vi "ELVIS III v1.0 Reserve Channel List.vi"(7 "Allow multiple opens?":bool, 8 "error in (no error)":errorcluster, 10 "Channel Reservation List":T1, 11 "Owner":string) -> (0 "error out":errorcluster)   [LabVIEW 2021]
uses:
  <vilib>/myRIO/Common/Instrument Driver Framework/ELVIS III v1.0/Resource Manager/typedefs/ELVIS III v1.0 Channel Reservation List.ctl
  <vilib>/myRIO/Common/Instrument Driver Framework/ELVIS III v1.0/Resource Manager/typedefs/ELVIS III v1.0 Channel Reservation Info.ctl
  <vilib>/myRIO/Common/Instrument Driver Framework/ELVIS III v1.0/Resource Manager/typedefs/ELVIS III v1.0 Connector List.ctl
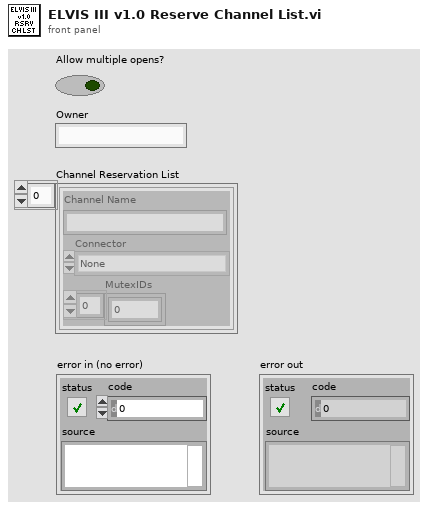
[diagram p1: front panel]
types:
  T1 = typedef "ELVIS III v1.0 Channel Reservation List.ctl" = T2[]
  T2 = typedef "ELVIS III v1.0 Channel Reservation Info.ctl" = cluster{"Channel Name":string, "Connector":T3, "MutexIDs":u32[]}
  T3 = typedef "ELVIS III v1.0 Connector List.ctl" = enum32{"None", "ConnectorA", "ConnectorB"}
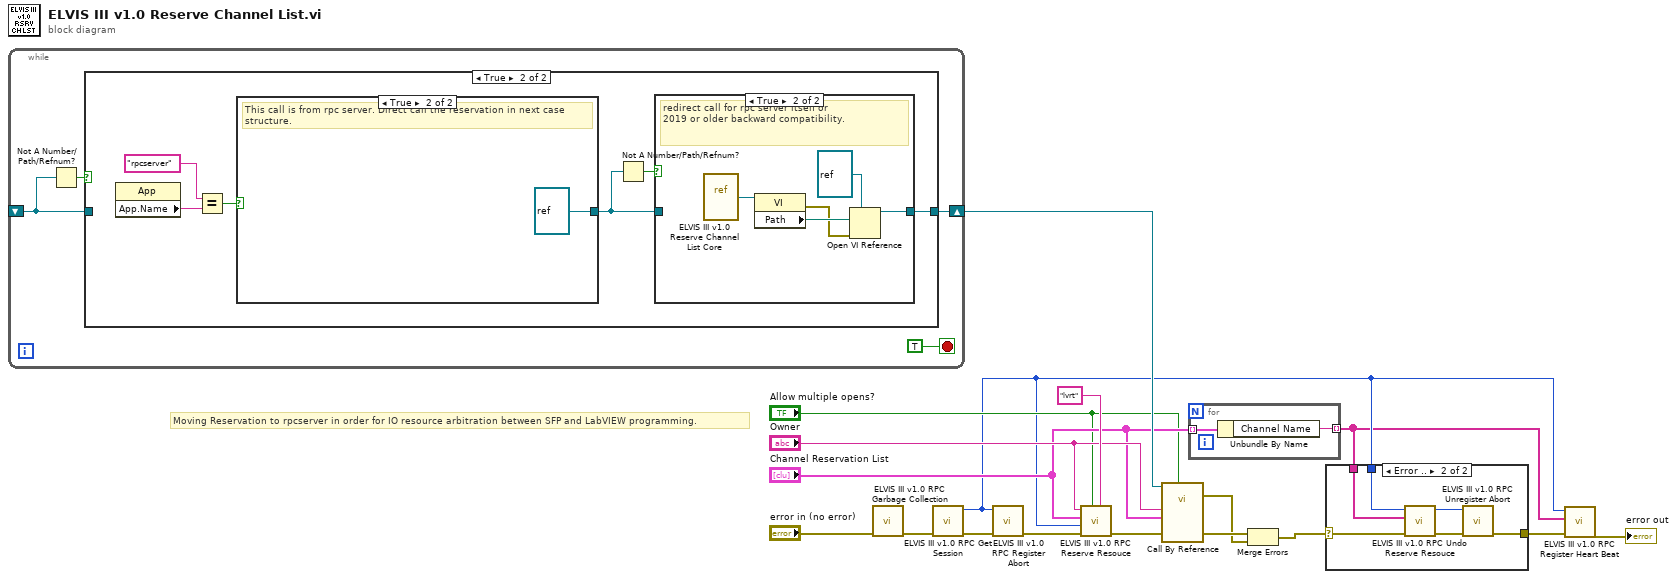
[diagram p0: block diagram]
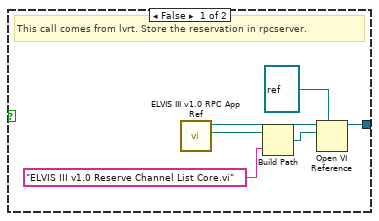
[diagram p5: hidden frame]
diagram:
  # "Moving Reservation to rpcserver in order for IO resource arbitration between SFP and LabVIEW programming."
  n1 = while {
    shift-right: [w21] -> w17
    shift-left: _ -> [w18]
    stop <- TRUE stop-if-true
    n2 = Not A Number/Path/Refnum?(number/path/refnum=w18) -> (NaN/Path/Refnum?=w19:bool)
    n3 = case shown="True" w19 {
      tunnel: [w22 w23] -> w21
      tunnel: w18 -> [w22 _]
      frame False {
      }
      frame True {
        n4 = property class="App"() -> ("App.Name"=w28:string)  [unwired: 2 in, 2 out]
        n5 = Equal?(x="rpcserver" ("Application:Name"), y=w28) -> (x = y?=w27:bool)
        n6 = case shown="True" w27 {
          tunnel: [w39 refnum<vi> refnum ("type specifier VI Refnum (for type only)")] -> w24
          frame False {
            # "This call comes from lvrt. Store the reservation in rpcserver."
            n7 = call <vilib>:"ELVIS III v1.0 RPC App Ref.vi"() -> ("Lib Path"=w37:path, "RPC Reference"=w38:refnum<vi>)  [unwired: 10 in]
            n8 = Build Path(base path=w37, name or relative path="ELVIS III v1.0 Reserve Channel List Core.vi") -> (appended path=w36:path)
            n9 = Open VI Reference(type specifier VI Refnum (for type only)=refnum<vi> refnum, application reference (local)=w38, vi path=w36) -> (vi reference=w39:refnum<vi>)  [unwired: 3 in, 1 out]
          }
          frame True {
            # "This call is from rpc server. Direct call the reservation in next case structure."
          }
        }
        n10 = Not A Number/Path/Refnum?(number/path/refnum=w24) -> (NaN/Path/Refnum?=w25:bool)
        n11 = case shown="True" w25 {
          tunnel: w24 -> [w29 _]
          tunnel: [w29 w32] -> w23
          frame False {
          }
          frame True {
            # "redirect call for rpc server itself or\n2019 or older backward compatibility."
            n12 = vi-ref <vilib>:"ELVIS III v1.0 Reserve Channel List Core.vi"() -> (w34:refnum<vi>)
            n13 = property class="VI"(reference=w34) -> (error out=w31:errorcluster, "Path"=w33:path)  [unwired: 1 in, 1 out]
            n14 = Open VI Reference(type specifier VI Refnum (for type only)=refnum<vi> refnum, vi path=w33, error in (no error)=w31) -> (vi reference=w32:refnum<vi>)  [unwired: 3 in, 1 out]
          }
        }
      }
    }
  }
  n15 = call <vilib>:"ELVIS III v1.0 RPC Garbage Collection.vi"("error in (no error)"="error in (no error)") -> ("error out"=w9:errorcluster)  [unwired: 10 in]
  n16 = call <vilib>:"ELVIS III v1.0 RPC Get Session.vi"("error in (no error)"=w9) -> ("error out"=w8:errorcluster, "Session"=w2:u32)  [unwired: 9 in]
  n17 = call <vilib>:"ELVIS III v1.0 RPC Register Abort.vi"("error in (no error)"=w8, "Session"=w2) -> ("error out"=w7:errorcluster)  [unwired: 9 in]
  n18 = call <vilib>:"ELVIS III v1.0 RPC Reserve Resouce.vi"("Owning Instrument"="lvrt", "Allow multiple opens?"="Allow multiple opens?", "error in (no error)"=w7, "Session"=w2, "Channel Reservation List"="Channel Reservation List", "Owner"="Owner") -> ("error out"=w6:errorcluster)  [unwired: 5 in]
  n19 = call-by-ref "?"(reference=w17, "Allow multiple opens?"="Allow multiple opens?", "error in (no error)"=w6, "Channel Reservation List"="Channel Reservation List", "Owner"="Owner") -> (error out=w4:errorcluster, 0:"error out"=w5:errorcluster)  [unwired: 8 in, 1 out]
  n20 = for {
    tunnel: "Channel Reservation List" -> [w43] mode=indexing
    tunnel: [w42] -> w1 mode=indexing
    n21 = Unbundle By Name(w43) -> ("Channel Name"=w42:string)
  }
  n22 = Merge Errors(w5, w4) -> (w3:errorcluster)
  n23 = case shown="Error .." w3 {
    selector: w3 -> [w44 w48]
    tunnel: [w44 w49] -> w10
    tunnel: w2 -> [_ w46]
    tunnel: w1 -> [_ w45]
    frame No Error {
    }
    frame Error {
      n24 = call <vilib>:"ELVIS III v1.0 RPC Undo Reserve Resouce.vi"("error in (no error)"=w48, "Channel Names"=w45, "Session"=w46) -> ("error out"=w47:errorcluster)  [unwired: 8 in]
      n25 = call <vilib>:"ELVIS III v1.0 RPC Unregister Abort.vi"("error in (no error)"=w47, "Session"=w46) -> ("error out"=w49:errorcluster)  [unwired: 9 in]
    }
  }
  n26 = call <vilib>:"ELVIS III v1.0 RPC Register Heart Beat.vi"("error in (no error)"=w10, "Channel Names"=w1, "Session"=w2) -> ("error out"=→"error out":errorcluster)  [unwired: 8 in]
